vi "Font Dialog__FD__LCR.vi"(8 "error in (no error)":errorcluster, 10 "Color In":u32, 11 "Font In":T1) -> (0 "error out":errorcluster, 2 "Color Out":u32, 3 "Font Out":T1)   [LabVIEW 2011, in "BooleanXControl__LCR.xctl"]
uses:
  BooleanXControl__LCR.xctl
panel:
  in  "Shadow":bool
  out "Desciption":string
  in  "Cancel":bool
  in  "OK":bool
  out "Preview":string
  in  "Size":i32
  in  "Color":u32(colorbox)
  in  "Outline":bool
  in  "Strikeout":bool
  in  "Underline":bool
  in  "Italic":bool
  in  "Bold":bool
  in  "Font":u16(ring) items=["6px2bus", "ACaslonPro-Bold", "ACaslonPro-BoldItalic", "ACaslonPro-Italic", "ACaslonPro-Regular", "ACaslonPro-Semibold", "ACaslonPro-SemiboldItalic", "AGaramondPro-Bold", "AGaramondPro-BoldItalic", "AGaramondPro-Italic", "AGaramondPro-Regular", "AdobeArabic-Bold", "AdobeArabic-BoldItalic", "AdobeArabic-Italic", "AdobeArabic-Regular", "AdobeFanHeitiStd-Bold", "AdobeFangsongStd-Regular", "AdobeGothicStd-Bold", "AdobeHebrew-Bold", "AdobeHebrew-BoldItalic", "AdobeHebrew-Italic", "AdobeHebrew-Regular", "AdobeHeitiStd-Regular", "AdobeKaitiStd-Regular", "AdobeMingStd-Light", "AdobeMyungjoStd-Medium", "AdobeSongStd-Light", "Agency FB", "Agency FB Bold", "Aharoni Bold", "Algerian", "Andalus", "Angsana New", "Angsana New Bold", "Angsana New Bold Italic", "Angsana New Italic", "AngsanaUPC", "AngsanaUPC Bold", "AngsanaUPC Bold Italic", "AngsanaUPC Italic", "Aparajita", "Aparajita Bold", "Aparajita Bold Italic(TrueType)", "Aparajita Italic", "Arabic Typesetting", "Arial", "Arial Black", "Arial Bold", "Arial Bold Italic", "Arial Italic", "Arial Narrow", "Arial Narrow Bold", "Arial Narrow Bold Italic", "Arial Narrow Italic", "Arial Rounded MT Bold", "Arial Unicode MS", "Baskerville Old Face", "Batang & BatangChe & Gungsuh & GungsuhChe", "Bauhaus 93", "Bell MT", "Bell MT Bold", "Bell MT Italic", "Berlin Sans FB", "Berlin Sans FB Bold", "Berlin Sans FB Demi Bold", "Bernard MT Condensed", "BirchStd", "Blackadder ITC", "BlackoakStd", "Bodoni MT", "Bodoni MT Black", "Bodoni MT Black Italic", "Bodoni MT Bold", "Bodoni MT Bold Italic", "Bodoni MT Condensed", "Bodoni MT Condensed Bold", "Bodoni MT Condensed Bold Italic", "Bodoni MT Condensed Italic", "Bodoni MT Italic", "Bodoni MT Poster Compressed", "Book Antiqua", "Book Antiqua Bold", "Book Antiqua Bold Italic", "Book Antiqua Italic", "Bookman Old Style", "Bookman Old Style Bold", "Bookman Old Style Bold Italic", "Bookman Old Style Italic", "Bookshelf Symbol 7", "Bradley Hand ITC", "Britannic Bold", "Broadway", "Browallia New", "Browallia New Bold", "Browallia New Bold Italic", "Browallia New Italic", "BrowalliaUPC", "BrowalliaUPC Bold", "BrowalliaUPC Bold Italic", "BrowalliaUPC Italic", "Brush Script MT Italic", "BrushScriptStd", "Calibri", "Calibri Bold", "Calibri Bold Italic", "Calibri Italic", "Californian FB", "Californian FB Bold", "Californian FB Italic", "Calisto MT", "Calisto MT Bold", "Calisto MT Bold Italic", "Calisto MT Italic", "Cambria & Cambria Math", "Cambria Bold", "Cambria Bold Italic", "Cambria Italic", "Candara", "Candara Bold", "Candara Bold Italic", "Candara Italic", "Castellar", "Centaur", "Century", "Century Gothic", "Century Gothic Bold", "Century Gothic Bold Italic", "Century Gothic Italic", "Century Schoolbook", "Century Schoolbook Bold", "Century Schoolbook Bold Italic", "Century Schoolbook Italic", "ChaparralPro-Bold", "ChaparralPro-BoldIt", "ChaparralPro-Italic", "ChaparralPro-Regular", "CharlemagneStd-Bold", "Chiller", "Colonna MT", "Comic Sans MS", "Comic Sans MS Bold", "Consolas", "Consolas Bold", "Consolas Bold Italic", "Consolas Italic", "Constantia", "Constantia Bold", "Constantia Bold Italic", "Constantia Italic", "Cooper Black", "CooperBlackStd", "CooperBlackStd-Italic", "Copperplate Gothic Bold", "Copperplate Gothic Light", "Corbel", "Corbel Bold", "Corbel Bold Italic", "Corbel Italic", "Cordia New", "Cordia New Bold", "Cordia New Bold Italic", "Cordia New Italic", "CordiaUPC", "CordiaUPC Bold", "CordiaUPC Bold Italic", "CordiaUPC Italic", "Courier 10,12,15", "Courier New", "Courier New Bold", "Courier New Bold Italic", "Courier New Italic", "Curlz MT", "DFKai-SB", "DaunPenh", "David", "David Bold", "DilleniaUPC", "DilleniaUPC Bold", "DilleniaUPC Bold Italic", "DilleniaUPC Italic", "DokChampa", "Ebrima", "Ebrima Bold", "Edwardian Script ITC", "Elephant", "Elephant Italic", "Engravers MT", "Eras Bold ITC", "Eras Demi ITC", "Eras Light ITC", "Eras Medium ITC", "Estrangelo Edessa", "EucrosiaUPC", "EucrosiaUPC Bold", "EucrosiaUPC Bold Italic", "EucrosiaUPC Italic", "Euphemia", "FZShuTi", "FZYaoTi", "FangSong", "Felix Titling", "Footlight MT Light", "Forte", "FrankRuehl", "Franklin Gothic Book", "Franklin Gothic Book Italic", "Franklin Gothic Demi", "Franklin Gothic Demi Cond", "Franklin Gothic Demi Italic", "Franklin Gothic Heavy", "Franklin Gothic Heavy Italic", "Franklin Gothic Medium", "Franklin Gothic Medium Cond", "Franklin Gothic Medium Italic", "FreesiaUPC", "FreesiaUPC Bold", "FreesiaUPC Bold Italic", "FreesiaUPC Italic", "Freestyle Script", "French Script MT", "Gabriola", "Garamond", "Garamond Bold", "Garamond Italic", "Gautami", "Gautami Bold", "Georgia", "Georgia Bold", "Georgia Bold Italic", "Georgia Italic", "GiddyupStd", "Gigi", "Gill Sans MT", "Gill Sans MT Bold", "Gill Sans MT Bold Italic", "Gill Sans MT Condensed", "Gill Sans MT Ext Condensed Bold", "Gill Sans MT Italic", "Gill Sans Ultra Bold", "Gill Sans Ultra Bold Condensed", "Gisha", "Gisha Bold", "Gloucester MT Extra Condensed", "Goudy Old Style", "Goudy Old Style Bold", "Goudy Old Style Italic", "Goudy Stout", "Gulim & GulimChe & Dotum & DotumChe", "Haettenschweiler", "Harlow Solid Italic", "Harrington", "High Tower Text", "High Tower Text Italic", "HoboStd", "Impact", "Imprint MT Shadow", "Informal Roman", "IrisUPC", "IrisUPC Bold", "IrisUPC Bold Italic", "IrisUPC Italic", "Iskoola Pota", "Iskoola Pota Bold", "JasmineUPC", "JasmineUPC Bold", "JasmineUPC Bold Italic", "JasmineUPC Italic", "Jokerman", "Juice ITC", "KaiTi", "Kalinga", "Kalinga Bold", "Kartika", "Kartika Bold", "Khmer UI", "Khmer UI Bold", "KodchiangUPC", "KodchiangUPC Bold", "KodchiangUPC Bold Italic", "KodchiangUPC Italic", "Kokila", "Kokila Bold", "Kokila Bold Italic(TrueType)", "Kokila Italic", "KozGoPr6N-Bold", "KozGoPr6N-ExtraLight", "KozGoPr6N-Heavy", "KozGoPr6N-Light", "KozGoPr6N-Medium", "KozGoPr6N-Regular", "KozGoPro-Bold", "KozGoPro-ExtraLight", "KozGoPro-Heavy", "KozGoPro-Light", "KozGoPro-Medium", "KozGoPro-Regular", "KozMinPr6N-Bold", "KozMinPr6N-ExtraLight", "KozMinPr6N-Heavy", "KozMinPr6N-Light", "KozMinPr6N-Medium", "KozMinPr6N-Regular", "KozMinPro-Bold", "KozMinPro-ExtraLight", "KozMinPro-Heavy", "KozMinPro-Light", "KozMinPro-Medium", "KozMinPro-Regular", "Kristen ITC", "Kunstler Script", "Lao UI", "Lao UI Bold", "Latha", "Latha Bold", "Leelawadee", "Leelawadee Bold", "LetterGothicStd", "LetterGothicStd-Bold", "LetterGothicStd-BoldSlanted", "LetterGothicStd-Slanted", "Levenim MT", "Levenim MT Bold", "LiSu", "LilyUPC", "LilyUPC Bold", "LilyUPC Bold Italic", "LilyUPC Italic", "LithosPro-Black", "LithosPro-Regular", "Lucida Bright", "Lucida Bright Demibold", "Lucida Bright Demibold Italic", "Lucida Bright Italic", "Lucida Calligraphy Italic", "Lucida Console", "Lucida Fax Demibold", "Lucida Fax Demibold Italic", "Lucida Fax Italic", "Lucida Fax Regular", "Lucida Handwriting Italic", "Lucida Sans Demibold Italic", "Lucida Sans Demibold Roman", "Lucida Sans Italic", "Lucida Sans Regular", "Lucida Sans Typewriter Bold", "Lucida Sans Typewriter Bold Oblique", "Lucida Sans Typewriter Oblique", "Lucida Sans Typewriter Regular", "Lucida Sans Unicode", "MS Gothic & MS PGothic & MS UI Gothic", "MS Mincho & MS PMincho", "MS Outlook", "MS Reference Sans Serif", "MS Reference Specialty", "MS Sans Serif 8,10,12,14,18,24", "MS Serif 8,10,12,14,18,24", "MT Extra", "MV Boli", "Magneto Bold", "Maiandra GD", "Malgun Gothic", "Malgun Gothic Bold", "Mangal", "Mangal Bold", "Matura MT Script Capitals", "Meiryo & Meiryo Italic & Meiryo UI & Meiryo UI Italic", "Meiryo Bold & Meiryo Bold Italic & Meiryo UI Bold & Meiryo UI Bold Italic", "MesquiteStd", "Microsoft Himalaya", "Microsoft JhengHei", "Microsoft JhengHei Bold", "Microsoft New Tai Lue", "Microsoft New Tai Lue Bold", "Microsoft PhagsPa", "Microsoft PhagsPa Bold", "Microsoft Sans Serif", "Microsoft Tai Le", "Microsoft Tai Le Bold", "Microsoft Uighur", "Microsoft YaHei", "Microsoft YaHei Bold", "Microsoft Yi Baiti", "MingLiU & PMingLiU & MingLiU_HKSCS", "MingLiU-ExtB & PMingLiU-ExtB & MingLiU_HKSCS-ExtB", "MinionPro-Bold", "MinionPro-BoldCn", "MinionPro-BoldCnIt", "MinionPro-BoldIt", "MinionPro-It", "MinionPro-Medium", "MinionPro-MediumIt", "MinionPro-Regular", "MinionPro-Semibold", "MinionPro-SemiboldIt", "Miriam", "Miriam Fixed", "Mistral", "Modern", "Modern No. 20", "Mongolian Baiti", "Monotype Corsiva", "MoolBoran", "MyriadPro-Bold", "MyriadPro-BoldCond", "MyriadPro-BoldCondIt", "MyriadPro-BoldIt", "MyriadPro-Cond", "MyriadPro-CondIt", "MyriadPro-It", "MyriadPro-Regular", "MyriadPro-Semibold", "MyriadPro-SemiboldIt", "Narkisim", "Niagara Engraved", "Niagara Solid", "NuevaStd-BoldCond", "NuevaStd-BoldCondItalic", "NuevaStd-Cond", "NuevaStd-CondItalic", "Nyala", "OCR A Extended", "OCRAStd", "Old English Text MT", "Onyx", "OratorStd", "OratorStd-Slanted", "Palace Script MT", "Palatino Linotype", "Palatino Linotype Bold", "Palatino Linotype Bold Italic", "Palatino Linotype Italic", "Papyrus", "Parchment", "Perpetua", "Perpetua Bold", "Perpetua Bold Italic", "Perpetua Italic", "Perpetua Titling MT Bold", "Perpetua Titling MT Light", "Plantagenet Cherokee", "Playbill", "Poor Richard", "PoplarStd", "PrestigeEliteStd-Bd", "Pristina", "Raavi", "Raavi Bold", "Rage Italic", "Ravie", "Rockwell", "Rockwell Bold", "Rockwell Bold Italic", "Rockwell Condensed", "Rockwell Condensed Bold", "Rockwell Extra Bold", "Rockwell Italic", "Rod", "Roman", "RosewoodStd-Regular", "STCaiyun", "STFangsong", "STHupo", "STKaiti", "STLiti", "STSong", "STXihei", "STXingkai", "STXinwei", "STZhongsong", "Sakkal Majalla", "Sakkal Majalla Bold", "Script", "Script MT Bold", "Segoe Print", "Segoe Print Bold", "Segoe Script", "Segoe Script Bold", "Segoe UI", "Segoe UI Bold", "Segoe UI Bold Italic", "Segoe UI Italic", "Segoe UI Light", "Segoe UI Semibold", "Segoe UI Symbol", "Shonar Bangla", "Shonar Bangla Bold", "Showcard Gothic", "Shruti", "Shruti Bold", "SimHei", "SimSun & NSimSun", "SimSun-ExtB", "Simplified Arabic", "Simplified Arabic Bold", "Simplified Arabic Fixed", "Small Fonts", "Small Fonts", "Snap ITC", "Stencil", "StencilStd", "Sylfaen", "Symbol", "Tahoma", "Tahoma Bold", "TektonPro-Bold", "TektonPro-BoldCond", "TektonPro-BoldExt", "TektonPro-BoldObl", "Tempus Sans ITC", "Times New Roman", "Times New Roman Bold", "Times New Roman Bold Italic", "Times New Roman Italic", "Traditional Arabic", "Traditional Arabic Bold", "TrajanPro-Bold", "TrajanPro-Regular", "Trebuchet MS", "Trebuchet MS Bold", "Trebuchet MS Bold Italic", "Trebuchet MS Italic", "Tunga", "Tunga Bold", "Tw Cen MT", "Tw Cen MT Bold", "Tw Cen MT Bold Italic", "Tw Cen MT Condensed", "Tw Cen MT Condensed Bold", "Tw Cen MT Condensed Extra Bold", "Tw Cen MT Italic", "Utsaah", "Utsaah Bold", "Utsaah Bold Italic(TrueType)", "Utsaah Italic", "Vani", "Vani Bold", "Verdana", "Verdana Bold", "Verdana Bold Italic", "Verdana Italic", "Vijaya", "Vijaya Bold", "Viner Hand ITC", "Vivaldi Italic", "Vladimir Script", "Vrinda", "Vrinda Bold", "Webdings", "Wide Latin", "Wingdings", "Wingdings 2", "Wingdings 3", "YouYuan"]
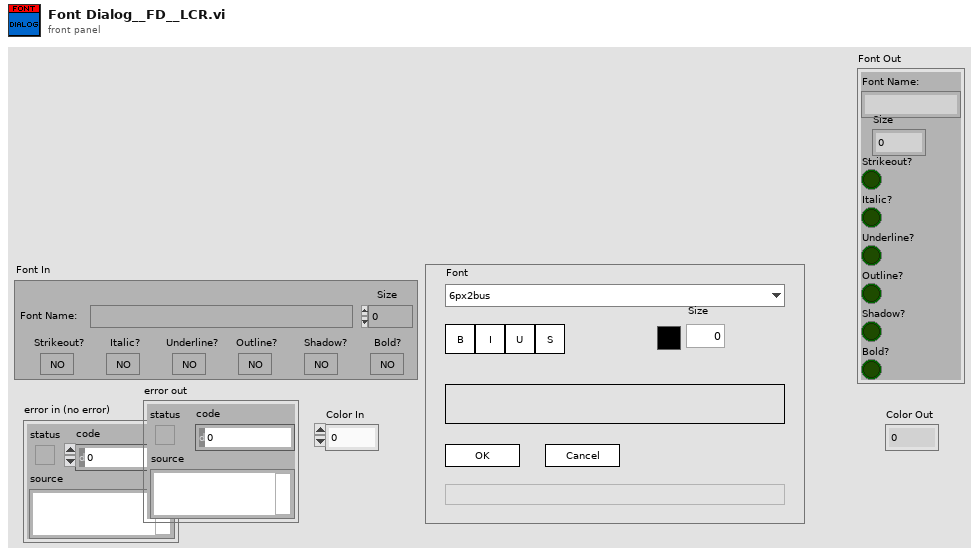
[diagram p1: front panel]
types:
  T1 = cluster{"Font Name:":string, "Size":i16, "Strikeout?":bool, "Italic?":bool, "Underline?":bool, "Outline?":bool, "Shadow?":bool, "Bold?":bool}
  T2 = enum16{"_Quit_", "Init", "Idle", "Exit", "Update", "Error"}
  T3 = cluster{"Font Name":string, "Size":u16, "Bold":bool, "Italic":bool, "Underline":bool, "Strikeout":bool, "Color":u32}
  T4 = typedef "lveventtype.ctl" = enum32{"Null", "Timeout", "App Instance Close", "App Instance Close?", "Autoscale Range Change", "Cell Edit", "Cell Edit?", "Cursor Grab", "Cursor Grab?", "Cursor Move", "Cursor Release", "Data Change", "Direction Change", "Display State Change", "Drag Ended", "Drag Enter", "Drag Leave", "Drag Over", "Drag Source Update", "Drag Starting", "Drag Starting?", "Drop", "Exec State Change", "Key Down", "Key Down?", "Key Repeat", "Key Repeat?", "Key Up", "Listbox Double Click", "Menu Activation?", "Menu Selection (App)", "Menu Selection? (App)", "Menu Selection (User)", "Mouse Down", "Mouse Down?", "Mouse Enter", "Mouse Leave", "Mouse Move", "Mouse Up", "NI Security User Change (App)", "Pane Size", "Panel Close", "Panel Close?", "Panel Resize", "Plot Attribute Change", "Scale Range Change", "Shortcut Menu Activation?", "Shortcut Menu Selection (App)", "Shortcut Menu Selection? (App)", "Shortcut Menu Selection (User)", "Tree Double Click", "Tree Drag", "Tree Drag?", "Tree Drop", "Tree Drop?", "Tree Item Close", "Tree Item Close?", "Tree Item Open", "Tree Item Open?", "Value Change"}
  T5 = typedef "eventvkey.ctl" = enum16{"ASCII", "Enter", "Return", "Shift", "Ctrl", "Alt", "Cmd", "Opt", "Caps", "NumLock", "Clear", "Break", "Up", "Down", "Left", "Right", "Insert", "Delete", "Home", "End", "PageUp", "PageDown", "Escape", "Help", "Pause", "ScrollLock", "F1", "F2", "F3", "F4", "F5", "F6", "F7", "F8", "F9", "F10", "F11", "F12", "F13", "F14", "F15", "F16", "F17", "F18", "F19", "F20", "F21", "F22", "F23", "F24", "Play", "VolumeUp", "VolumeDown", "Mute", "Two Byte Char"}
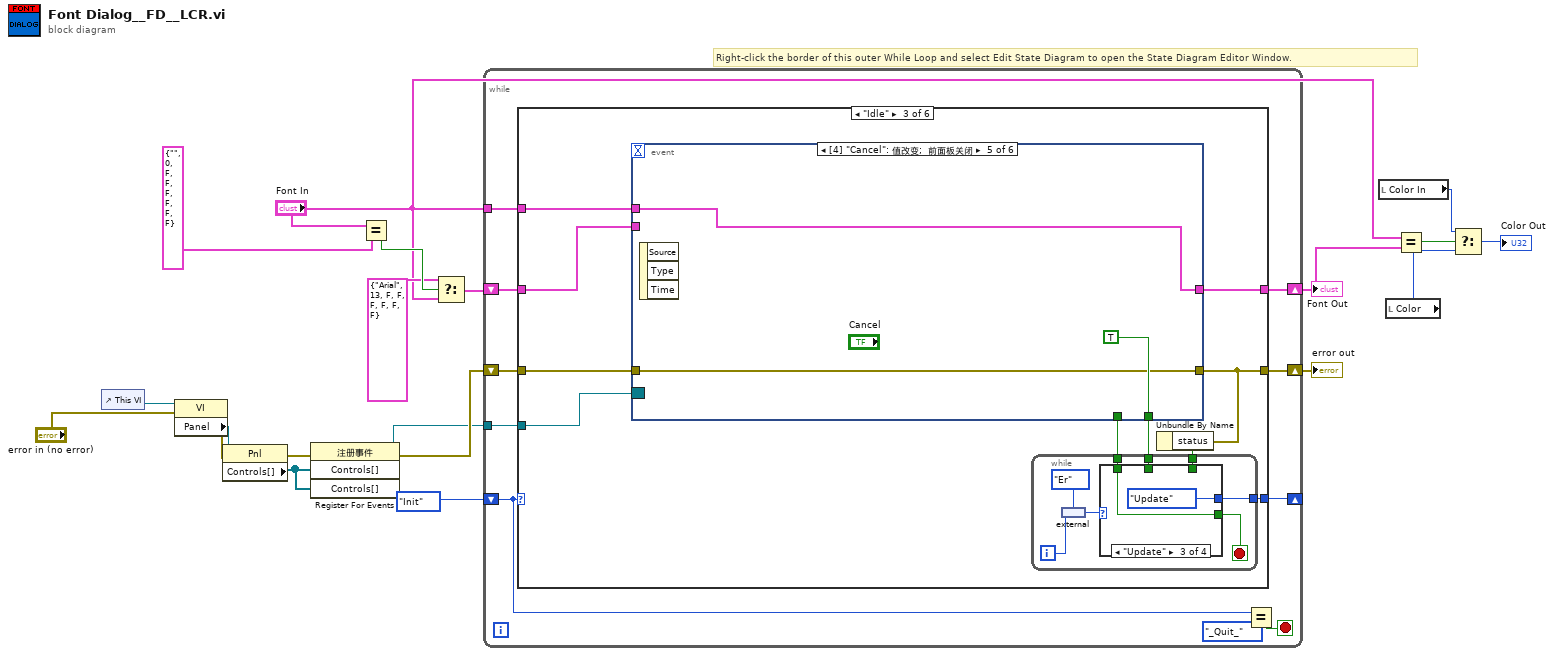
[diagram p0: block diagram]
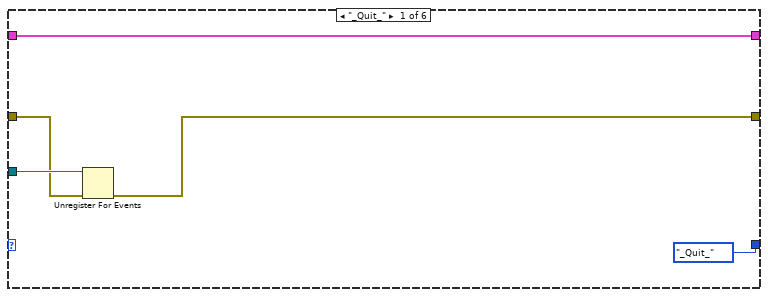
[diagram p2: hidden frame]
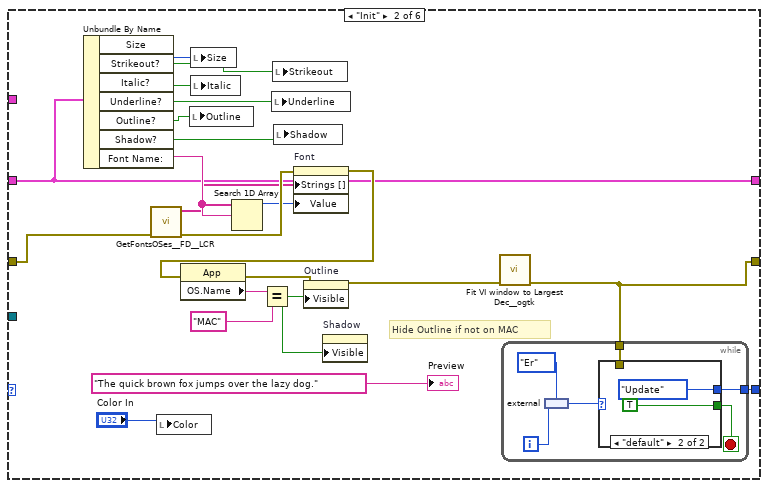
[diagram p3: hidden frame]
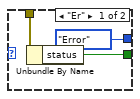
[diagram p4: hidden frame]
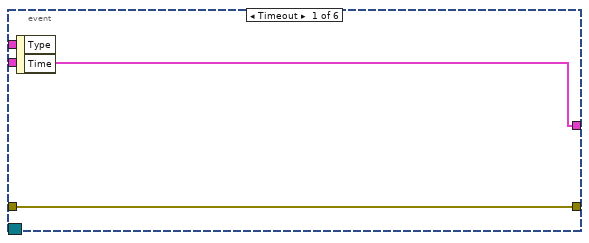
[diagram p5: hidden frame]
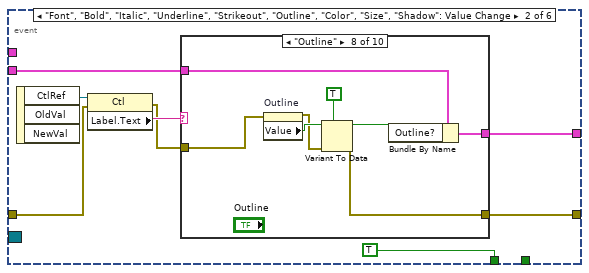
[diagram p6: hidden frame]
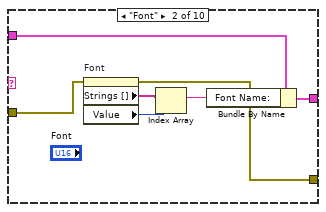
[diagram p8: hidden frame]
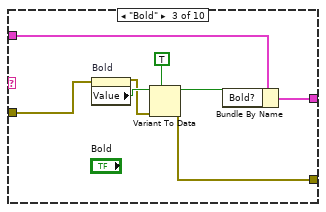
[diagram p9: hidden frame]
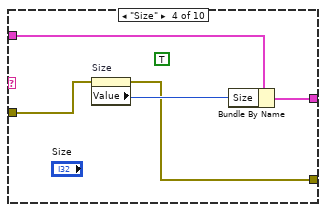
[diagram p10: hidden frame]
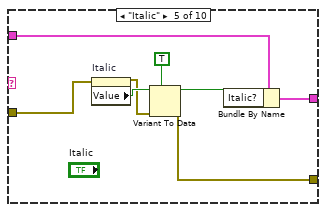
[diagram p11: hidden frame]
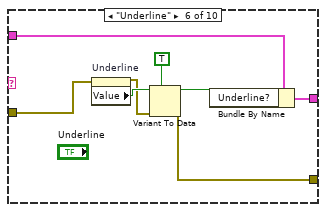
[diagram p12: hidden frame]
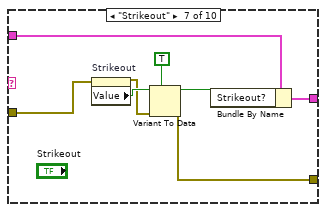
[diagram p13: hidden frame]
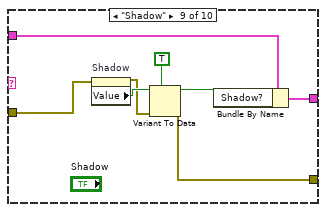
[diagram p14: hidden frame]
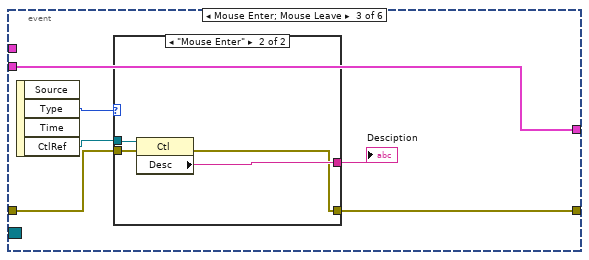
[diagram p16: hidden frame]
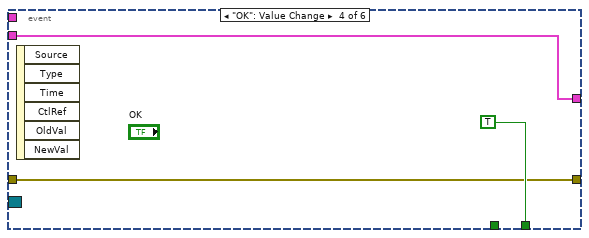
[diagram p18: hidden frame]
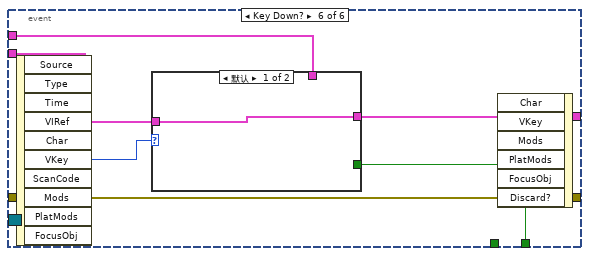
[diagram p19: hidden frame]
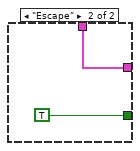
[diagram p20: hidden frame]
diagram:
  # "Right-click the border of this outer While Loop and select Edit State Diagram to open the State Diagram Editor Window."
  n1 = control-ref of="This VI"() -> (w15:refnum<vi>)
  n2 = property class="VI"(reference=w15, error in="error in (no error)") -> (error out=w14:errorcluster, "Panel"=w13:refnum<vi>)  [unwired: 1 out]
  n3 = property class="Pnl"(reference=w13, error in=w14) -> (error out=w12:errorcluster, "Controls[]"=w10:refnum<vi>[])  [unwired: 1 out]
  n4 = register-events(error in=w12, w10, w10) -> (reference out=w8:refnum<event-registration>, error out=w9:errorcluster)  [unwired: 1 in]
  n5 = Equal?(x="Font In", y=T1 {"Font Name:"="", "Size"=0, "Strikeout?"=FALSE, "Italic?"=FALSE, "Underline?"=FALSE, "Outline?"=FALSE, "Shadow?"=FALSE, "Bold?"=FALSE} ("Font In")) -> (x = y?=w18:bool)
  n6 = Select(t=T1 {"Font Name:"="Arial", "Size"=13, "Strikeout?"=FALSE, "Italic?"=FALSE, "Underline?"=FALSE, "Outline?"=FALSE, "Shadow?"=FALSE, "Bold?"=FALSE} ("Font In"), s=w18, f="Font In") -> (s? t:f=w17:T1)
  n7 = while {
    shift-right: [w29] -> _
    shift-left: T2."Init" -> [w30]
    tunnel: "Font In" -> [w26]
    shift-right: [w25] -> w5
    shift-left: w17 -> [w24]
    shift-right: [w22] -> w7
    shift-left: w9 -> [w23]
    tunnel: w8 -> [w21]
    stop <- w28 stop-if-true
    n8 = case shown="\"Idle\"" w30 {
      tunnel: [T2."_Quit_" w57 w83 w207 w232 w251] -> w29
      tunnel: w26 -> [_ _ w77 _ _ w250]
      tunnel: [w34 w37 w80 w206 w221 w250] -> w25
      tunnel: w24 -> [w34 w37 w81 w206 w221 _]
      tunnel: w23 -> [w32 w48 w82 w205 w223 w249]
      tunnel: [w31 w50 w74 w205 w220 w249] -> w22
      tunnel: w21 -> [w33 _ w76 _ _ _]
      frame "_Quit_" {
        n9 = Unregister For Events(event registration refnum=w33, error in=w32) -> (error out=w31:errorcluster)
      }
      frame "Init" {
        # "Hide Outline if not on MAC"
        n10 = Unbundle By Name(w37) -> ("Size"=w43:i16, "Strikeout?"=w42:bool, "Italic?"=w41:bool, "Underline?"=w40:bool, "Outline?"=w39:bool, "Shadow?"=w38:bool, "Font Name:"=w47:string)
        n11 = call "GetFontsOSes__FD__LCR.vi"("error in (no error)"=w48) -> ("error out"=w46:errorcluster, "SystemFonts"=w45:string[])  [unwired: 9 in]
        n12 = local write "Color"("Color In") -> ()
        n13 = local write "Outline"(w39) -> ()
        n14 = local write "Size"(w43) -> ()
        n15 = local write "Italic"(w41) -> ()
        n16 = Search 1D Array(1D array=w45, element=w47) -> (index of element=w44:i32)  [unwired: 1 in]
        n17 = local write "Underline"(w40) -> ()
        n18 = local write "Strikeout"(w42) -> ()
        n19 = local write "Shadow"(w38) -> ()
        n20 = property on="Font" class="Ring (严格)"(error in=w46, "Strings []"=w45, "Value"=w44) -> (error out=w49:errorcluster)  [unwired: 1 in, 1 out]
        n21 = property class="App"(error in=w49) -> (error out=w54:errorcluster, "OS.Name"=w56:string)  [unwired: 1 in, 1 out]
        n22 = Equal?(x=w56, y="MAC") -> (x = y?=w52:bool)
        n23 = property on="Outline" class="Bool (严格)"(error in=w54, "Visible"=w52) -> (error out=w51:errorcluster)  [unwired: 1 in, 1 out]
        n24 = property on="Shadow" class="Bool (严格)"("Visible"=w52) -> ()  [unwired: 2 in, 2 out]
        n25 = call <userlib>:"Fit VI window to Largest Dec__ogtk.vi"("error in (no error)"=w51) -> ("error out"=w50:errorcluster)  [unwired: 5 in, 1 out]
        n26 = while {
          tunnel: [w60] -> w57
          tunnel: w50 -> [w58]
          i -> [w63]
          stop <- w59 stop-if-true
          n27 = external ("Integer to Enum")(enum16{"Er", "default"}."Er", w63) -> (w61:enum16{"Er", "default"})
          n28 = case shown="\"default\"" w61 {
            tunnel: [T2."Error" T2."Update"] -> w60
            tunnel: [w69 TRUE] -> w59
            tunnel: w58 -> [w70 _]
            frame "Er" {
              n29 = Unbundle By Name(w70) -> ("status"=w69:bool)
            }
            frame "default" {
            }
          }
        }
        "Preview" <- "The quick brown fox jumps over the lazy dog."
      }
      frame "Idle" {
        n30 = event shown="[4] \"Cancel\": 值改变;  前面板关闭" {
          selector: w76 -> [_ _ _ _ _ _]
          dyn-events: _ -> [_ _ _ _ _ _]
          timeout: _ -> [_ _ _ _ _ _]
          tunnel: w82 -> [w84 w92 w161 w169 w173 w179]
          tunnel: w81 -> [w85 w89 w158 w171 _ w175]
          tunnel: [w85 w88 w158 w171 w172 w176] -> w80
          tunnel: [_ TRUE _ _ _ _] -> w79
          tunnel: [w84 w86 w159 w169 w173 w179] -> w74
          tunnel: [_ _ _ TRUE TRUE w180] -> w78
          tunnel: w77 -> [_ _ _ _ w172 w177]
          event Timeout {
            n31 = event-data() -> ()  [unwired: 1 in, 2 out]
          }
          event "Font", "Bold", "Italic", "Underline", "Strikeout", "Outline", "Color", "Size", "Shadow": Value Change {
            n32 = event-data() -> ("CtlRef"=w93:refnum<vi>)  [unwired: 1 in, 2 out]
            n33 = property class="Ctl"(reference=w93, error in=w92) -> (error out=w90:errorcluster, "Label.Text"=w91:string)  [unwired: 1 out]
            n34 = case shown="\"Outline\"" w91 {
              tunnel: w90 -> [w94 w102 w110 w115 w123 w131 w139 w147 w155 w156]
              tunnel: w89 -> [w95 w98 w109 w114 w122 w130 w138 w146 w154 w157]
              tunnel: [w95 w97 w108 w113 w121 w129 w137 w145 w153 w157] -> w88
              tunnel: [w94 w96 w103 w111 w116 w124 w132 w140 w148 w156] -> w86
              frame "False", Default {
              }
              frame "Font" {
                n35 = property on="Font" class="Ring (严格)"(error in=w102) -> (error out=w96:errorcluster, "Strings []"=w101:string[], "Value"=w100:u16)  [unwired: 1 in, 1 out]
                n36 = Index Array(array=w101, index=w100) -> (element=w99:string)
                n37 = Bundle By Name(cluster=w98, "Font Name:"=w99) -> (w97:T1)
              }
              frame "Bold" {
                n38 = property on="Bold" class="Bool (严格)"(error in=w110) -> (error out=w104:errorcluster, "Value"=w107:bool)  [unwired: 1 in, 1 out]
                n39 = Variant To Data(error in=w104, type=TRUE, Variant=w107) -> (data=w106:bool, error out=w103:errorcluster)
                n40 = Bundle By Name(cluster=w109, "Bold?"=w106) -> (w108:T1)
              }
              frame "Size" {
                (unwired) TRUE
                n41 = property on="Size" class="DigNum (严格)"(error in=w115) -> (error out=w111:errorcluster, "Value"=w112:i32)  [unwired: 1 in, 1 out]
                n42 = Bundle By Name(cluster=w114, "Size"=w112) -> (w113:T1)
              }
              frame "Italic" {
                n43 = property on="Italic" class="Bool (严格)"(error in=w123) -> (error out=w117:errorcluster, "Value"=w120:bool)  [unwired: 1 in, 1 out]
                n44 = Variant To Data(error in=w117, type=TRUE, Variant=w120) -> (data=w119:bool, error out=w116:errorcluster)
                n45 = Bundle By Name(cluster=w122, "Italic?"=w119) -> (w121:T1)
              }
              frame "Underline" {
                n46 = property on="Underline" class="Bool (严格)"(error in=w131) -> (error out=w125:errorcluster, "Value"=w128:bool)  [unwired: 1 in, 1 out]
                n47 = Variant To Data(error in=w125, type=TRUE, Variant=w128) -> (data=w127:bool, error out=w124:errorcluster)
                n48 = Bundle By Name(cluster=w130, "Underline?"=w127) -> (w129:T1)
              }
              frame "Strikeout" {
                n49 = property on="Strikeout" class="Bool (严格)"(error in=w139) -> (error out=w133:errorcluster, "Value"=w136:bool)  [unwired: 1 in, 1 out]
                n50 = Variant To Data(error in=w133, type=TRUE, Variant=w136) -> (data=w135:bool, error out=w132:errorcluster)
                n51 = Bundle By Name(cluster=w138, "Strikeout?"=w135) -> (w137:T1)
              }
              frame "Outline" {
                n52 = property on="Outline" class="Bool (严格)"(error in=w147) -> (error out=w141:errorcluster, "Value"=w144:bool)  [unwired: 1 in, 1 out]
                n53 = Variant To Data(error in=w141, type=TRUE, Variant=w144) -> (data=w143:bool, error out=w140:errorcluster)
                n54 = Bundle By Name(cluster=w146, "Outline?"=w143) -> (w145:T1)
              }
              frame "Shadow" {
                n55 = property on="Shadow" class="Bool (严格)"(error in=w155) -> (error out=w149:errorcluster, "Value"=w152:bool)  [unwired: 1 in, 1 out]
                n56 = Variant To Data(error in=w149, type=TRUE, Variant=w152) -> (data=w151:bool, error out=w148:errorcluster)
                n57 = Bundle By Name(cluster=w154, "Shadow?"=w151) -> (w153:T1)
              }
              frame "Color" {
              }
            }
          }
          event Mouse Enter; Mouse Leave {
            n58 = event-data() -> ("Type"=w163:T4, "CtlRef"=w162:refnum<vi>)  [unwired: 1 in, 2 out]
            n59 = case shown="\"Mouse Enter\"" w163 {
              tunnel: w162 -> [_ w168]
              tunnel: w161 -> [w164 w167]
              tunnel: [_ w166] -> w160
              tunnel: [w164 w165] -> w159
              frame Default {
              }
              frame "Mouse Enter" {
                n60 = property class="Ctl"(reference=w168, error in=w167) -> (error out=w165:errorcluster, "Desc"=w166:string)  [unwired: 1 out]
              }
            }
            "Desciption" <- w160
          }
          event "OK": Value Change {
            n61 = event-data() -> ()  [unwired: 1 in, 6 out]
          }
          event "Cancel": Value Change; Panel Close {
            n62 = event-data() -> ()  [unwired: 1 in, 3 out]
          }
          event Key Down? {
            n63 = event-data() -> ("VKey"=w178:T5)  [unwired: 1 in, 9 out]
            n64 = case shown="默认" w178 {
              tunnel: [_ TRUE] -> w180
              tunnel: [w181 w182] -> w176
              tunnel: w177 -> [_ w182]
              tunnel: w175 -> [w181 _]
              frame Default {
              }
              frame "Escape" {
              }
            }
            n65 = event-data() -> ()  [unwired: 7 in, 1 out]
          }
        }
        n66 = Unbundle By Name(w74) -> ("status"=w75:bool)
        n67 = while {
          tunnel: [w188] -> w83
          tunnel: w79 -> [w186]
          tunnel: w78 -> [w185]
          tunnel: w75 -> [w184]
          i -> [w191]
          stop <- w187 stop-if-true
          n68 = external ("Integer to Enum")(enum16{"Er", "Exit", "Update", "default"}."Er", w191) -> (w189:enum16{"Er", "Exit", "Update", "default"})
          n69 = case shown="\"Update\"" w189 {
            tunnel: [T2."Error" T2."Exit" T2."Update" T2."Idle"] -> w188
            tunnel: [w197 w199 w201 TRUE] -> w187
            tunnel: w186 -> [_ _ w201 _]
            tunnel: w185 -> [_ w199 _ _]
            tunnel: w184 -> [w197 _ _ _]
            frame "Er" {
            }
            frame "Exit" {
            }
            frame "Update" {
            }
            frame "default" {
            }
          }
        }
      }
      frame "Exit" {
        n70 = while {
          tunnel: [w209] -> w207
          i -> [w212]
          stop <- w208 stop-if-true
          n71 = external ("Integer to Enum")(enum16{"default"}."default", w212) -> (w210:enum16{"default"})
          n72 = case shown="\"default\"" w210 {
            tunnel: [T2."_Quit_"] -> w209
            tunnel: [TRUE] -> w208
            frame "default" {
            }
          }
        }
      }
      frame "Update" {
        n73 = Unbundle By Name(w221) -> ("Font Name:"=w230:string, "Size"=w229:i16, "Bold?"=w228:bool, "Italic?"=w227:bool, "Underline?"=w226:bool, "Strikeout?"=w225:bool)
        n74 = Bundle By Name(cluster=T3 {"Font Name"="", "Size"=0, "Bold"=FALSE, "Italic"=FALSE, "Underline"=FALSE, "Strikeout"=FALSE, "Color"=0} ("Text.Font"), "Font Name"=w230, "Size"=w229, "Bold"=w228, "Italic"=w227, "Underline"=w226, "Strikeout"=w225, "Color"="Color") -> (w222:T3)
        n75 = property on="Preview" class="Str"(error in=w223, "Text.Font"=w222) -> (error out=w220:errorcluster)  [unwired: 1 in, 1 out]
        n76 = while {
          tunnel: [w235] -> w232
          tunnel: w220 -> [w233]
          i -> [w238]
          stop <- w234 stop-if-true
          n77 = external ("Integer to Enum")(enum16{"Er", "default"}."Er", w238) -> (w236:enum16{"Er", "default"})
          n78 = case shown="\"Er\"" w236 {
            tunnel: [T2."Error" T2."Idle"] -> w235
            tunnel: [w245 TRUE] -> w234
            tunnel: w233 -> [w244 _]
            frame "Er" {
              n79 = Unbundle By Name(w244) -> ("status"=w245:bool)
            }
            frame "default" {
            }
          }
        }
      }
      frame "Error" {
        n80 = while {
          tunnel: [w253] -> w251
          i -> [w256]
          stop <- w252 stop-if-true
          n81 = external ("Integer to Enum")(enum16{"default"}."default", w256) -> (w254:enum16{"default"})
          n82 = case shown="\"default\"" w254 {
            tunnel: [T2."Exit"] -> w253
            tunnel: [TRUE] -> w252
            frame "default" {
            }
          }
        }
      }
    }
    n83 = Equal?(x=w30, y=T2."_Quit_") -> (x = y?=w28:bool)
  }
  "Font Out" <- w5
  "error out" <- w7
  n84 = local read "Color In"() -> (w3:u32)
  n85 = local read "Color"() -> (w2:u32)
  n86 = Equal?(x="Font In", y=w5) -> (x = y?=w4:bool)
  n87 = Select(t=w3, s=w4, f=w2) -> (s? t:f=→"Color Out":u32)
